vi "DB read & write data type.vi"(6 "read/write":u16(ring) items=["Read", "Write"], 11 "Part setup":T1) -> ()   [LabVIEW 2015]
uses:
  Control 1.ctl
panel:
  # "First motor testing Parameter"
  # "Printing Info"
  # "Second motor testing Parameter"
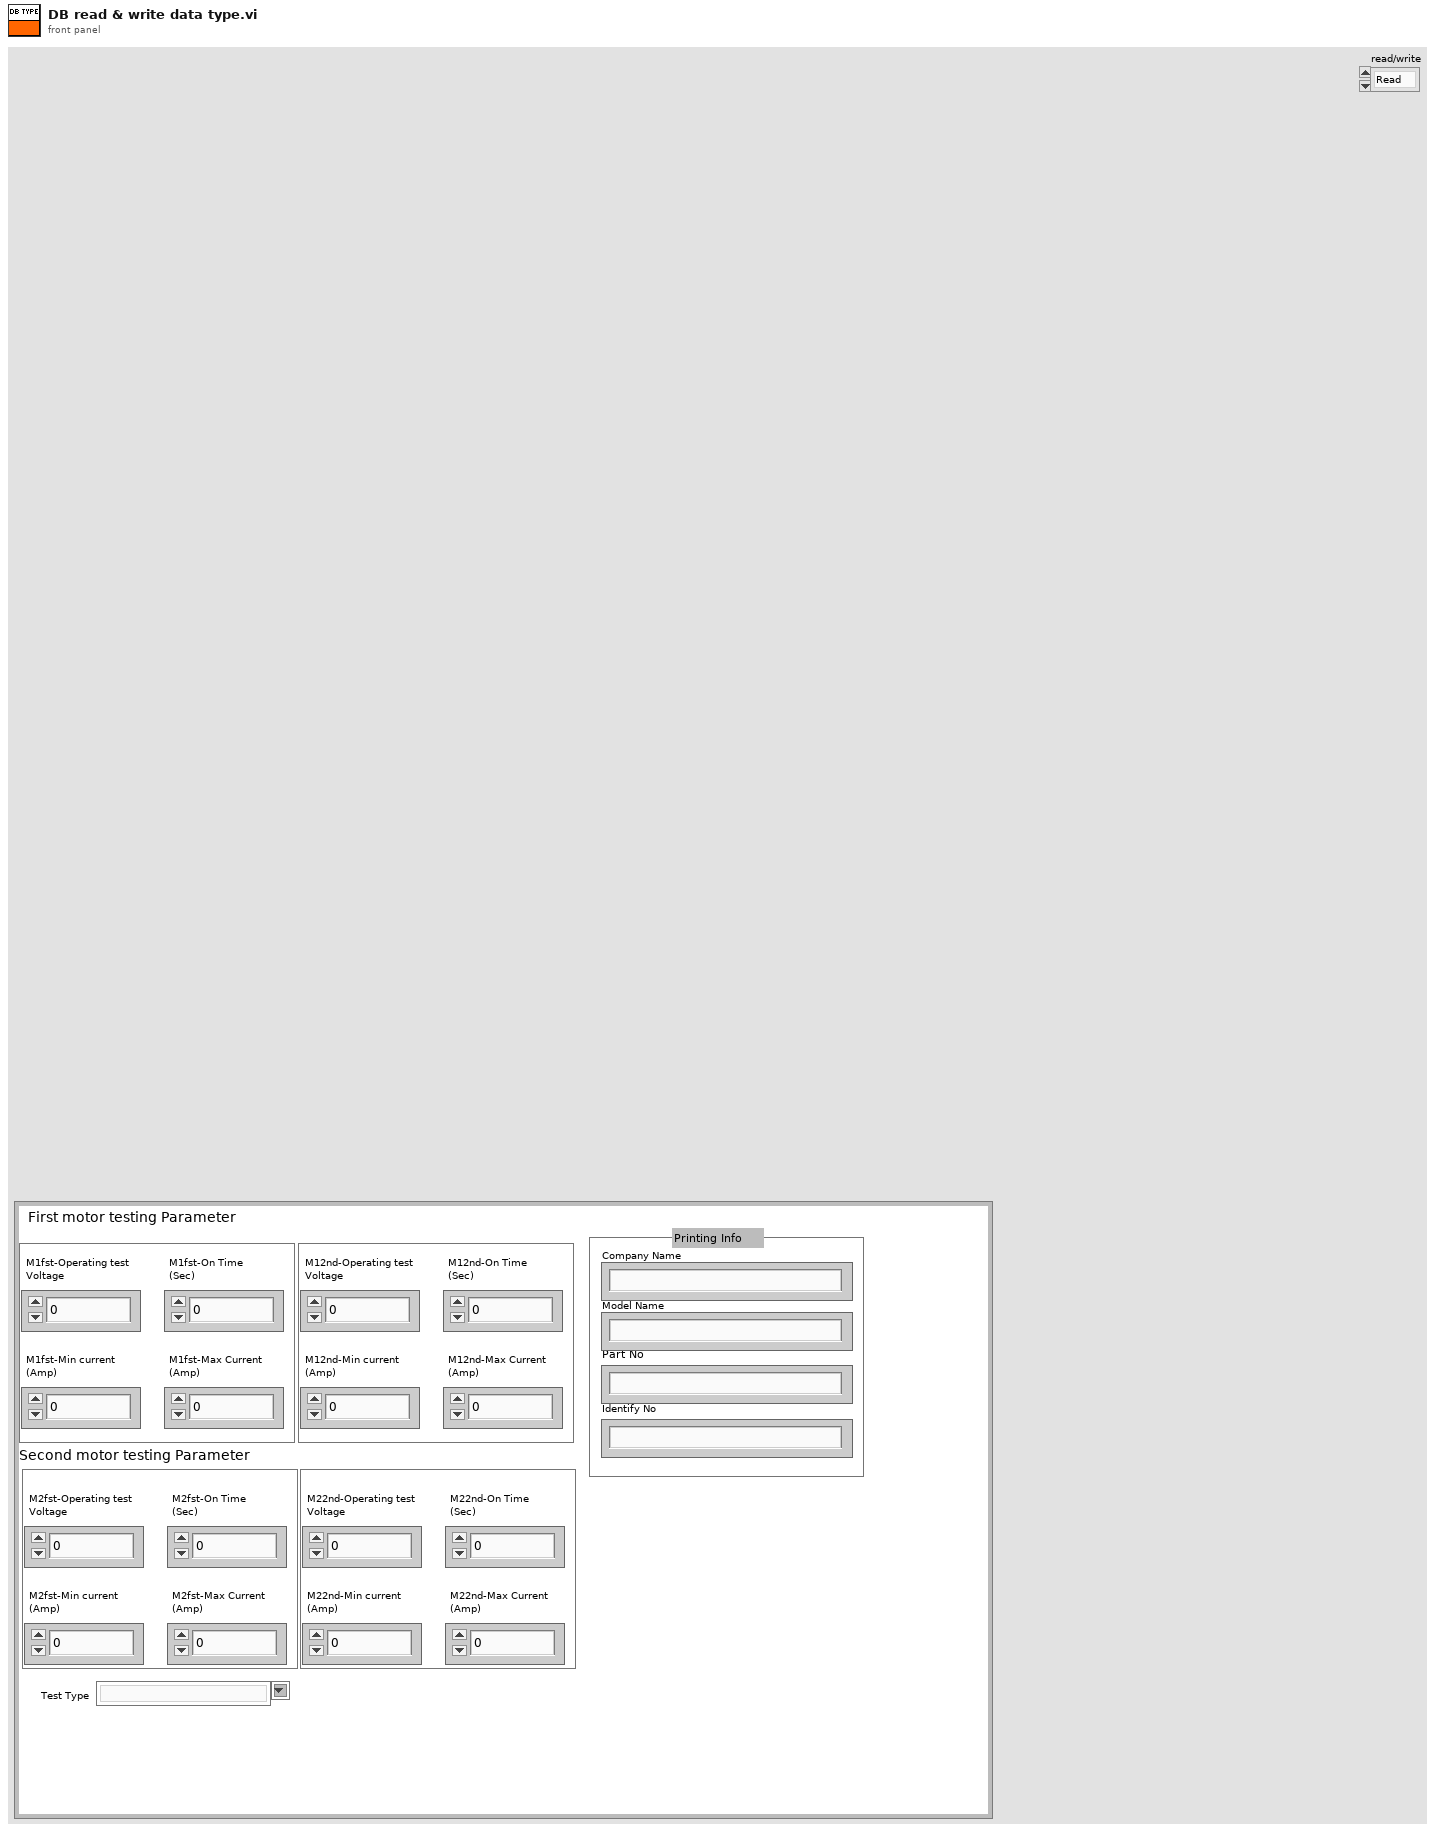
[diagram p1: front panel]
types:
  T1 = typedef "Control 1.ctl" = cluster{"Model Name":string, "Company Name":string, "Part No":string, "Identify No":string, "M1fst-Operating test\nVoltage":dbl, "M1fst-On Time \n(Sec)":dbl, "M1fst-Min current \n(Amp)":dbl, "M1fst-Max Current\n(Amp)":dbl, "M12nd-Operating test\nVoltage":dbl, "M12nd-On Time \n(Sec)":dbl, "M12nd-Min current \n(Amp)":dbl, "M12nd-Max Current\n(Amp)":dbl, "M2fst-Operating test\nVoltage":dbl, "M2fst-On Time \n(Sec)":dbl, "M2fst-Min current \n(Amp)":dbl, "M2fst-Max Current\n(Amp)":dbl, "M22nd-Operating test\nVoltage":dbl, "M22nd-On Time \n(Sec)":dbl, "M22nd-Min current \n(Amp)":dbl, "M22nd-Max Current\n(Amp)":dbl, "Test Type ":string}
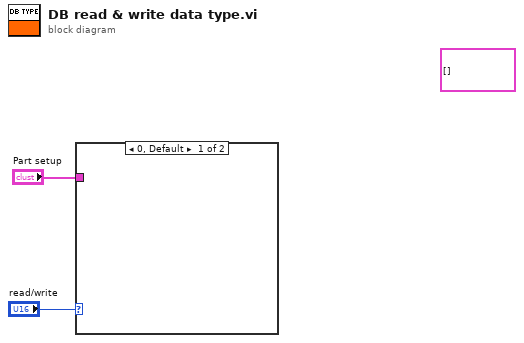
[diagram p0: block diagram]
diagram:
  (unwired) T1[] []
  n1 = case shown="0, Default" "read/write" {
    tunnel: "Part setup" -> [_ _]
    frame 0, Default {
    }
    frame 1 {
    }
  }
